vi "DrawSubMenuRectangle.vi"(7 "Collection in":refnum<class "Collection.lvclass">, 8 "error in (no error)":errorcluster, 10 "Area":T1, 11 "Menu in":refnum<class "Menu.lvclass">) -> (0 "error out":errorcluster, 2 "Area":T1, 3 "Menu out":refnum<class "Menu.lvclass">, 5 "Collection out":refnum<class "Collection.lvclass">)   [LabVIEW 2021, in "Menu.lvlib" / "Menu.lvclass"]
uses:
  Menu.lvclass
  Menu.lvclass/Menu.ctl
  Picture2D/src/Collection/Collection.lvclass
  Picture2D/src/Rectangle/Rectangle.lvclass
  Picture2D/src/PointSpecialized/PointSpecialized.lvclass
  C:/GitHub/Picture2D/src/Point/Point.lvclass
  C:/GitHub/Picture2D/src/IDrawable/IDrawable.lvclass
  C:/GitHub/Picture2D/src/IMovable/IMovable.lvclass
  C:/GitHub/Picture2D/src/IRotatable/IRotatable.lvclass
  C:/GitHub/Picture2D/src/IScalable/IScalable.lvclass
  C:/GitHub/Picture2D/src/PointSpecialized/PointSpecialized.lvclass
  C:/GitHub/Picture2D/src/Polygone/Polygone.lvclass
  C:/GitHub/Picture2D/src/Shape/Shape.lvclass
  C:/GitHub/Picture2D/src/Picture2D/Picture2D.lvclass
  C:/GitHub/Picture2D/src/Rectangle/Rectangle.lvclass
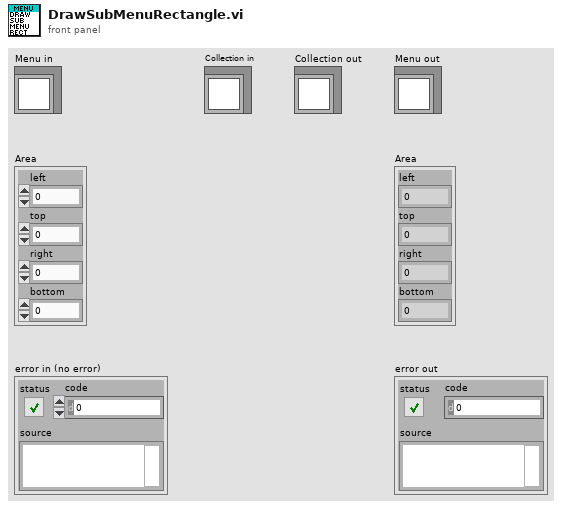
[diagram p1: front panel]
types:
  T1 = cluster{"left":i16, "top":i16, "right":i16, "bottom":i16}
  T2 = typedef "Menu.lvlib/Menu.lvclass/MenuColors.ctl" = cluster{"Text":refnum<class "Color.lvclass">, "HiliteText":refnum<class "Color.lvclass">, "Background":refnum<class "Color.lvclass">, "BorderColor":refnum<class "Color.lvclass">, "Hilite":refnum<class "Color.lvclass">}
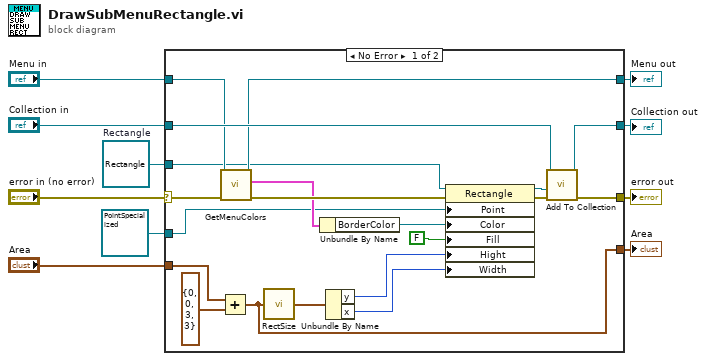
[diagram p0: block diagram]
diagram:
  w1 = refnum<class "Rectangle.lvclass"> refnum  # Rectangle
  n1 = case shown="No Error" "error in (no error)" {
    selector: "error in (no error)" -> [w18 w32]
    tunnel: [w30 w32] -> w10
    tunnel: [w28 w33] -> w8
    tunnel: [w19 w31] -> w7
    tunnel: "Area" -> [w22 w31]
    tunnel: "Collection in" -> [w21 w33]
    tunnel: "Menu in" -> [w15 w34]
    tunnel: [w16 w34] -> w3
    tunnel: refnum<class "PointSpecialized.lvclass"> refnum ("Point") -> [w13 _]
    tunnel: w1 -> [w12 _]
    frame No Error {
      n2 = Add(x=w22, y=T1 {"left"=0, "top"=0, "right"=3, "bottom"=3} ("Area")) -> (x+y=w19:T1)
      n3 = call "GetMenuColors.vi"("error in (no error)"=w18, "Menu in"=w15) -> ("error out"=w17:errorcluster, "MenuColors"=w14:T2, "Menu out"=w16:refnum<class "Menu.lvclass">)  [unwired: 7 in]
      n4 = call <vilib>:"RectSize.vi"("rect"=w19) -> ("point"=w24:cluster{"x":i16, "y":i16})
      n5 = Unbundle By Name(w14) -> ("BorderColor"=w11:refnum<class "Color.lvclass">)
      n6 = Unbundle By Name(w24) -> ("y"=w25:i16, "x"=w26:i16)
      n7 = property class="Rectangle"(reference=w12, error in=w17, "Point"=w13, "Color"=w11, "Fill"=FALSE, "Hight"=w25, "Width"=w26) -> (reference out=w27:refnum<class "Rectangle.lvclass">, error out=w29:errorcluster)
      n8 = call-dynamic "Add To Collection.vi"("error in (no error)"=w29, "IDrawable"=w27, "Collection in"=w21) -> ("error out"=w30:errorcluster, "Collection out"=w28:refnum<class "Collection.lvclass">)  [unwired: 7 in]
    }
    frame Error {
    }
  }
  "error out" <- w10
  "Collection out" <- w8
  "Area" <- w7
  "Menu out" <- w3
